vi "Find rotated points.vi"(7 "Axis reference":u32, 9 "Line seg \nlength":u32, 10 "Angle (deg)":sgl, 11 "Origin":cluster{"X":sgl, "Y":sgl}) -> (2 "Point Coordinates (y axis)":cluster{"X":dbl, "Y":dbl}, 3 "Point 1 coordinates (x axis)":cluster{"X":dbl, "Y":dbl})   [LabVIEW 2019]
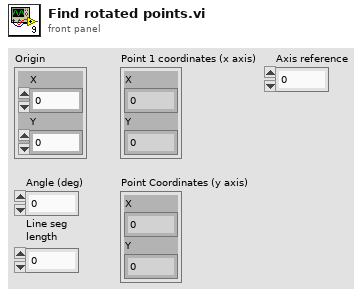
[diagram p1: front panel]
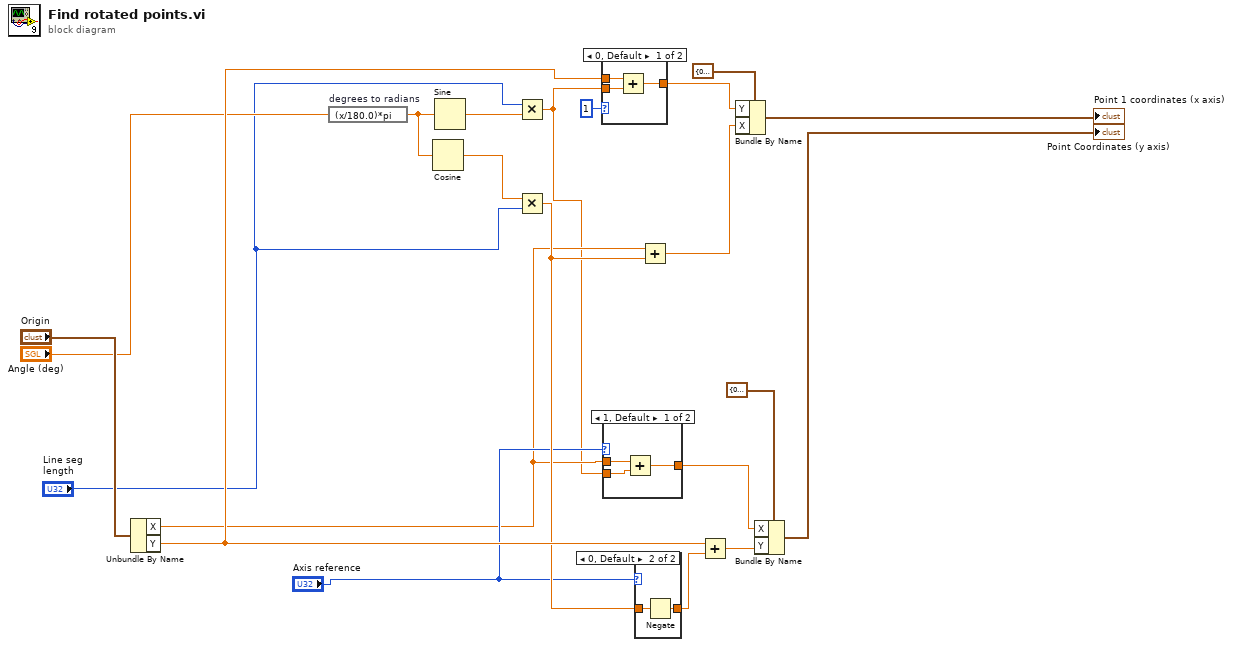
[diagram p0: block diagram]
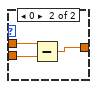
[diagram p2: hidden frame]
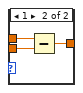
[diagram p3: hidden frame]
diagram:
  n1 = Unbundle By Name("Origin") -> ("X"=w3:sgl, "Y"=w20:sgl)
  n2 = expression code="(x/180.0)*pi" "degrees to radians"("Angle (deg)") -> (w8:sgl)
  n3 = Cosine(x=w8) -> (cos(x)=w9:sgl)
  n4 = Sine(x=w8) -> (sin(x)=w16:sgl)
  n5 = Multiply(x="Line seg \nlength", y=w16) -> (x*y=w2:sgl)
  n6 = Multiply(x=w9, y="Line seg \nlength") -> (x*y=w7:sgl)
  n7 = case shown="0, Default" u32 1 ("Axis reference") {
    tunnel: w20 -> [w24 w27]
    tunnel: w2 -> [w23 w26]
    tunnel: [w22 w25] -> w15
    frame 0, Default {
      n8 = Add(x=w24, y=w23) -> (x+y=w22:sgl)
    }
    frame 1 {
      n9 = Subtract(x=w27, y=w26) -> (x-y=w25:sgl)
    }
  }
  n10 = case shown="1, Default" "Axis reference" {
    tunnel: w3 -> [w30 w33]
    tunnel: w2 -> [w29 w32]
    tunnel: [w28 w31] -> w1
    frame 1, Default {
      n11 = Add(x=w30, y=w29) -> (x+y=w28:sgl)
    }
    frame 0 {
      n12 = Subtract(x=w33, y=w32) -> (x-y=w31:sgl)
    }
  }
  n13 = case shown="0, Default" "Axis reference" {
    tunnel: w7 -> [w34 w36]
    tunnel: [w34 w35] -> w6
    frame 1 {
    }
    frame 0, Default {
      n14 = Negate(x=w36) -> (-x=w35:sgl)
    }
  }
  n15 = Add(x=w3, y=w7) -> (x+y=w12:sgl)
  n16 = Add(x=w20, y=w6) -> (x+y=w14:sgl)
  n17 = Bundle By Name(cluster=cluster{"X":dbl, "Y":dbl} {"X"=0.0, "Y"=0.0} ("Point Coordinates"), "Y"=w15, "X"=w12) -> (→"Point 1 coordinates (x axis)":cluster{"X":dbl, "Y":dbl})
  n18 = Bundle By Name(cluster=cluster{"X":dbl, "Y":dbl} {"X"=0.0, "Y"=0.0} ("Point Coordinates"), "X"=w1, "Y"=w14) -> (→"Point Coordinates (y axis)":cluster{"X":dbl, "Y":dbl})
